vi "Create Picture Ring Code.vi"(8 "Panel Origin":T1, 9 "Object Data":T2, 10 "Ring Image Default Image":string, 11 "Ring Image Variable Name":string) -> (2 "JS Code For Indicators":string, 3 "HTML":string)   [LabVIEW 2015, in "Front Panel Publisher.lvlib" / "Select.lvclass"]
uses:
  Select.lvclass
  Object_class/Attributes.ctl
  Object_class/Coordinates.ctl
  <vilib>/Utility/miscctls.llb/LVPointTypeDef.ctl
  Front Panel Publisher.lvlib
  Object_class/Object.lvclass
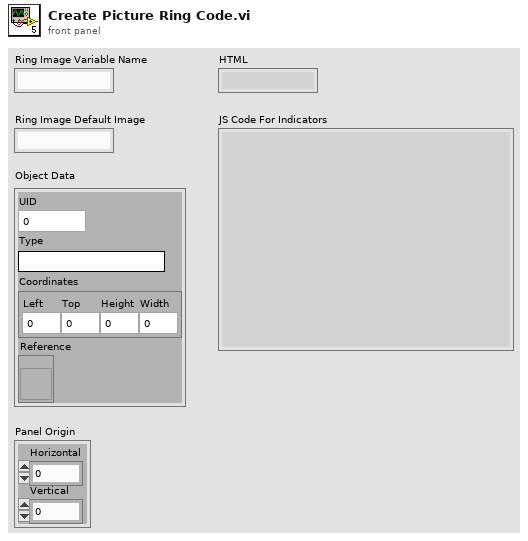
[diagram p1: front panel]
types:
  T1 = typedef "LVPointTypeDef.ctl" = cluster{"Horizontal":i16, "Vertical":i16}
  T2 = typedef "Front Panel Publisher.lvlib/Object.lvclass/Attributes.ctl" = cluster{"UID":i32, "Type":string, "Coordinates":T3, "Reference":refnum<vi>}
  T3 = typedef "Front Panel Publisher.lvlib/Object.lvclass/Coordinates.ctl" = cluster{"Left":i32, "Top":i32, "Height":u32, "Width":u32}
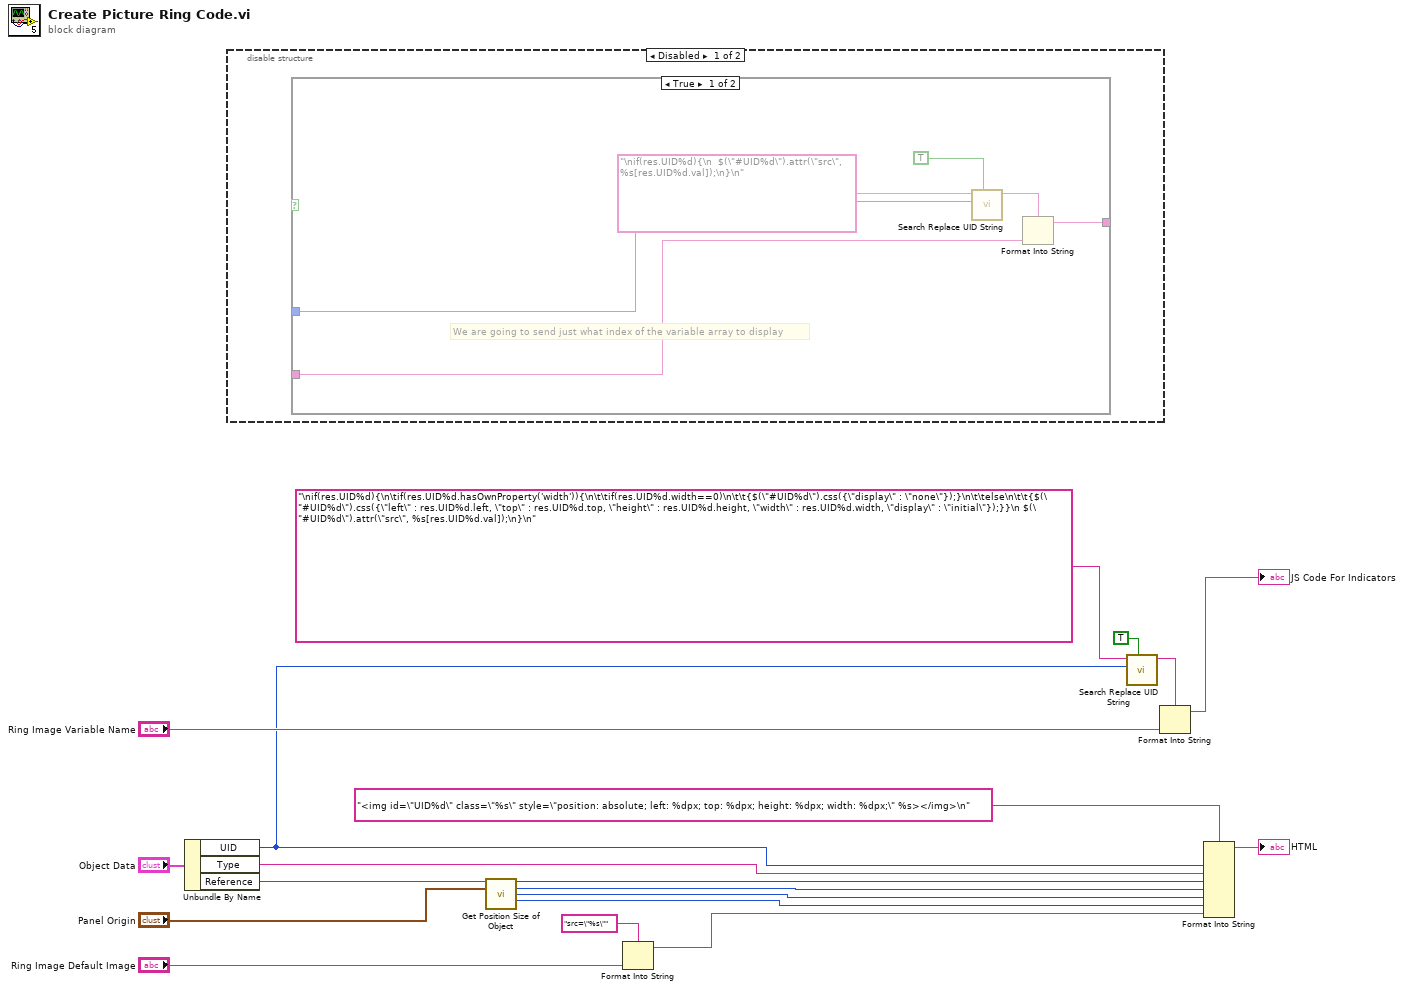
[diagram p0: block diagram]
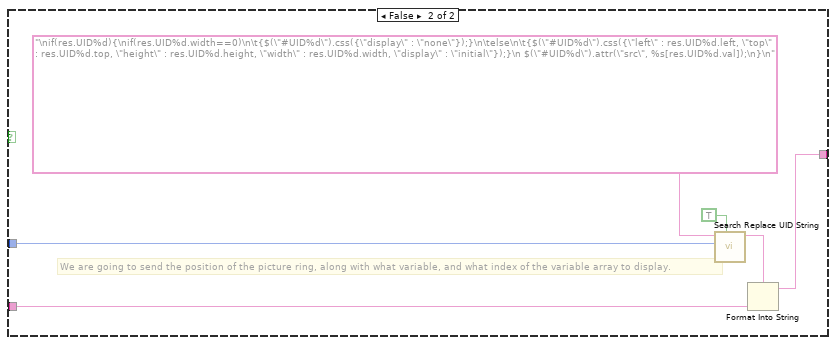
[diagram p2: hidden frame]
diagram:
  n1 = Unbundle By Name("Object Data") -> ("UID"=w14:i32, "Type"=w16:string, "Reference"=w9:refnum<vi>)
  n2 = disable-structure shown="Disabled" {
    frame Disabled {
      n3 = case shown="True" {
        selector: _ -> [_ _]
        tunnel: [w25 w31] -> _
        tunnel: _ -> [w24 w30]
        tunnel: _ -> [w22 w27]
        frame True {
          # "We are going to send just what index of the variable array to display"
          n4 = call "Search Replace UID String.vi"("Replace All Numeric Inputs"=TRUE, "UID"=w22, "Input String"="\nif(res.UID%d){\n  $(\"#UID%d\").attr(\"src\", %s[res.UID%d.val]);\n}\n") -> ("Output String"=w20:string)  [unwired: 8 in]
          n5 = Format Into String(format string=w20, w24) -> (resulting string=w25:string)  [unwired: 2 in, 1 out]
        }
        frame False {
          # "We are going to send the position of the picture ring, along with what variable, and what index of the variable array to display."
          n6 = call "Search Replace UID String.vi"("Replace All Numeric Inputs"=TRUE, "UID"=w27, "Input String"="\nif(res.UID%d){\nif(res.UID%d.width==0)\n\t{$(\"#UID%d\").css({\"display\" : \"none\"});}\n\telse\n\t{$(\"#UID%d\").css({\"left\" : res.UID%d.left, \"top\" : res.UID%d.top, \"height\" : res.UID%d.height, \"width\" : res.UID%d.width, \"display\" : \"initial\"});}\n $(\"#UID%d\").attr(\"src\", %s[res.UID%d.val]);\n}\n") -> ("Output String"=w26:string)  [unwired: 8 in]
          n7 = Format Into String(format string=w26, w30) -> (resulting string=w31:string)  [unwired: 2 in, 1 out]
        }
      }
    }
    frame Enabled {
    }
  }
  n8 = call "Get Position Size of Object.vi"("GObject in"=w9, "Panel Origin"="Panel Origin") -> ("Left"=w8:i32, "Top"=w7:i32, "Height"=w6:u32, "Width"=w5:u32)  [unwired: 9 in, 1 out]
  n9 = Format Into String(format string="src=\"%s\"", "Ring Image Default Image") -> (resulting string=w12:string)  [unwired: 2 in, 1 out]
  n10 = call "Search Replace UID String.vi"("Replace All Numeric Inputs"=TRUE, "UID"=w14, "Input String"="\nif(res.UID%d){\n\tif(res.UID%d.hasOwnProperty('width')){\n\t\tif(res.UID%d.width==0)\n\t\t{$(\"#UID%d\").css({\"display\" : \"none\"});}\n\t\telse\n\t\t{$(\"#UID%d\").css({\"left\" : res.UID%d.left, \"top\" : res.UID%d.top, \"height\" : res.UID%d.height, \"width\" : res.UID%d.width, \"display\" : \"initial\"});}}\n $(\"#UID%d\").attr(\"src\", %s[res.UID%d.val]);\n}\n") -> ("Output String"=w2:string)  [unwired: 8 in]
  n11 = Format Into String(format string=w2, "Ring Image Variable Name") -> (resulting string=→"JS Code For Indicators":string)  [unwired: 2 in, 1 out]
  n12 = Format Into String(format string="<img id=\"UID%d\" class=\"%s\" style=\"position: absolute; left: %dpx; top: %dpx; height: %dpx; width: %dpx;\" %s></img>\n", w14, w16, w8, w7, w6, w5, w12) -> (resulting string=→"HTML":string)  [unwired: 2 in, 1 out]
